vi "Test_UnfilledBuffer_AvgEquals0.vi"(8 "error in (no error)":errorcluster, 11 "TestCase in":refnum<class "TestTimedAverageBuffer.lvclass">) -> (0 "error out":errorcluster, 3 "TestCase out":refnum<class "TestTimedAverageBuffer.lvclass">)   [LabVIEW 2015, in "TestTimedAverageBuffer.lvclass"]
uses:
  TestTimedAverageBuffer.lvclass
  TimedAverageBuffer.lvclass/TimedAverageBuffer.ctl
  <vilib>/Utility/High Resolution Relative Seconds.vi
  <vilib>/addons/_JKI Toolkits/VI Tester/TestCase.llb/TestCase.lvclass
  TimedAverageBuffer.lvclass
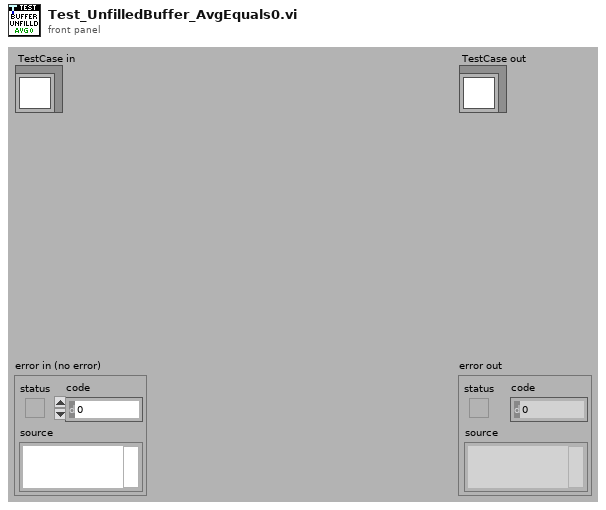
[diagram p1: front panel]
types:
  T1 = typedef "TimedAverageBuffer.lvlib/TimedAverageBuffer.lvclass/TimedAverageBuffer Reference.ctl" = refnum<data-value>
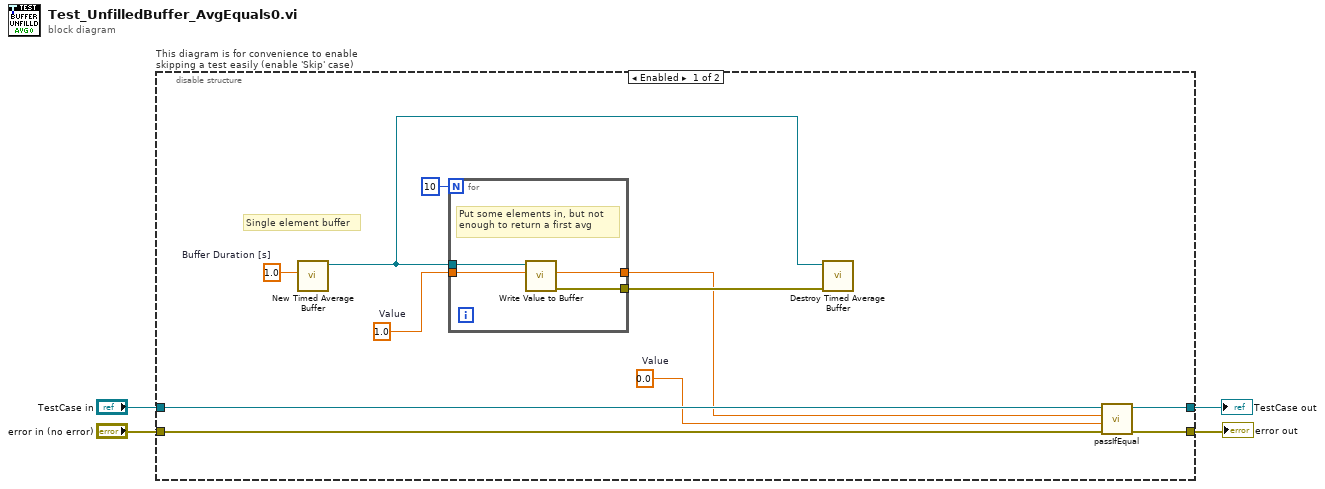
[diagram p0: block diagram]
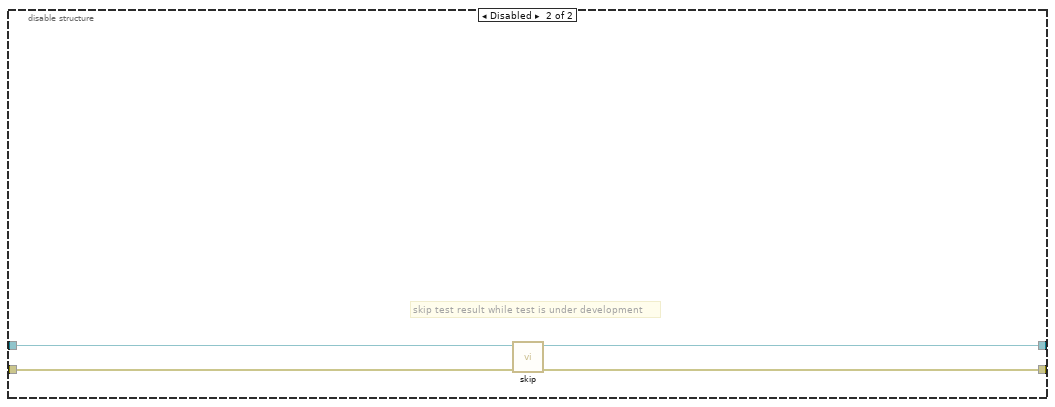
[diagram p2: hidden frame]
diagram:
  n1 = disable-structure "This diagram is for convenience to enable skipping a test easily (enable 'Skip' case)" shown="Enabled" {
    disable-tunnel: "TestCase in" -> [w15 w23]
    disable-tunnel: [w14 w21] -> w1
    disable-tunnel: [w13 w22] -> w3
    disable-tunnel: "error in (no error)" -> [w12 w20]
    frame Enabled {
      w6 = 0.0  # Value
      w5 = 1.0  # Buffer Duration [s]
      w8 = 1.0  # Value
      # "Single element buffer"
      n2 = call "New Timed Average Buffer.vi"("Buffer Duration [s]"=w5) -> ("Timed Average Buffer"=w11:T1)  [unwired: 9 in, 1 out]
      n3 = for {
        N: 10 -> [_]
        tunnel: w11 -> [w19]
        tunnel: [w18] -> w10
        tunnel: [w16] -> w9
        tunnel: w8 -> [w17]
        # "Put some elements in, but not\nenough to return a first avg"
        n4 = call "Write Value to Buffer.vi"("Value"=w17, "Timed Average Buffer"=w19) -> ("error out"=w18:errorcluster, "Average"=w16:dbl)  [unwired: 6 in, 2 out]
      }
      n5 = call "Destroy Timed Average Buffer.vi"("error in (no error)"=w10, "Timed Average Buffer"=w11) -> ()  [unwired: 9 in, 1 out]
      n6 = call-dynamic "passIfEqual.vi"("error in (no error)"=w12, "y"=w6, "x"=w9, "TestCase in"=w15) -> ("error out"=w13:errorcluster, "TestCase out"=w14:refnum<class "TestTimedAverageBuffer.lvclass">)  [unwired: 6 in]
    }
    frame Disabled {
      # "skip test result while test is under development"
      n7 = call <vilib>:"skip.vi"("error in (no error)"=w20, "TestCase in"=w23) -> ("error out"=w22:errorcluster, "TestCase out"=w21:refnum<class "TestTimedAverageBuffer.lvclass">)  [unwired: 8 in]
    }
  }
  "error out" <- w3
  "TestCase out" <- w1
